vi "Last Ack.vi"(8 "error in (no error)":errorcluster, 11 "Queue in":refnum<queue>) -> ()   [LabVIEW 2018, in "EZ Message.lvlib"]
uses:
  EZ Message.lvlib
  Message.ctl
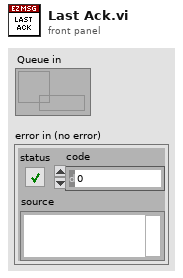
[diagram p1: front panel]
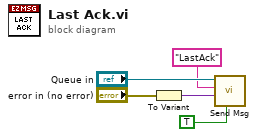
[diagram p0: block diagram]
diagram:
  n1 = To Variant(anything="error in (no error)") -> (Variant=w1:variant)
  n2 = call "Send Msg.vi"("Priority Message (F)"=TRUE, "Msg Value"=w1, "Msg Name"="LastAck", "Msg Queue In"="Queue in") -> ()  [unwired: 4 in, 4 out]
